vi "+S2C_VAR_Manager.vi"() -> ()   [LabVIEW 2015]
panel:
  in  "Array":T1(array[cluster])=[{"Name"="MyString", "Array"=["", "String"], "Tag"="MyString", "Indent"=0}, {"Name"="MyNumber", "Array"=["0", "Number"], "Tag"="MyNumber", "Indent"=0}, {"Name"="MyBoolean", "Array"=["False", "Boolean"], "Tag"="MyBoolean", "Indent"=0}, {"Name"="MyThis", "Array"=["", "String"], "Tag"="MyThis", "Indent"=0}, {"Name"="MyThat", "Array"=["", "String"], "Tag"="MyThat", "Indent"=0}, {"Name"="<Right-click for new variable>", "Array"=[], "Tag"="*New", "Indent"=0}]
  out "Init":bool
  out "Error Out":errorcluster
  in  "Error In":errorcluster
  in  "Table":string[](tree) caption="Variable Manager"
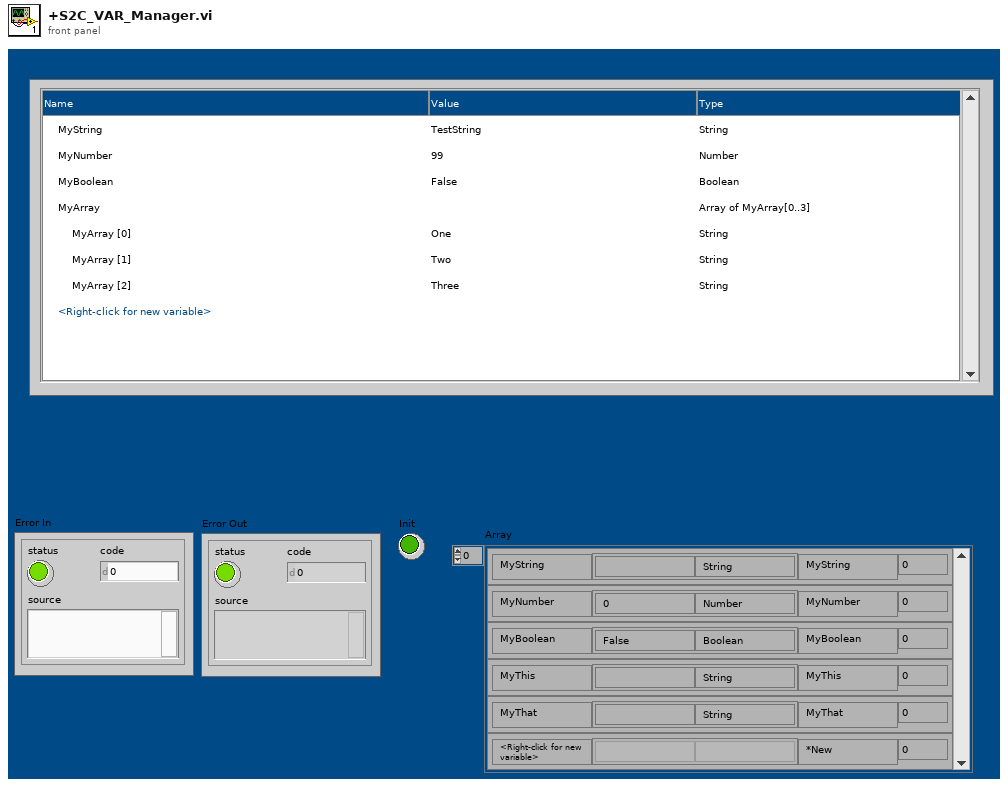
[diagram p1: front panel]
types:
  T1 = cluster{"Name":string, "Array":string[], "Tag":string, "Indent":i32}[]
  T2 = typedef "LVPoint32TypeDef.ctl" = cluster{"Horizontal":i32, "Vertical":i32}
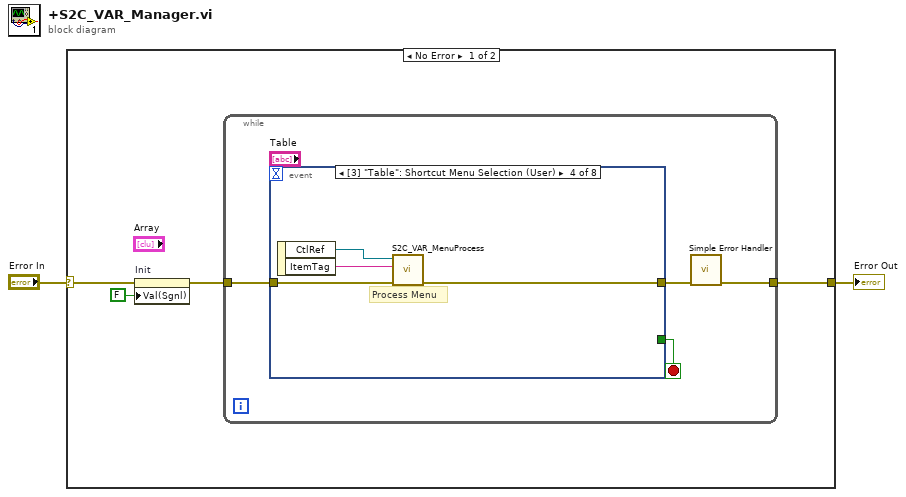
[diagram p0: block diagram]
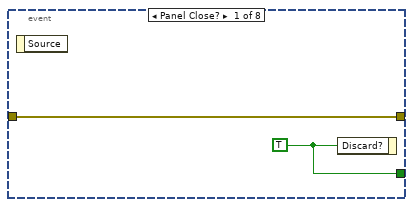
[diagram p2: hidden frame]
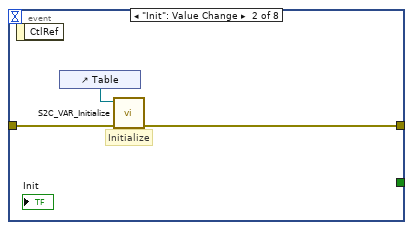
[diagram p3: hidden frame]
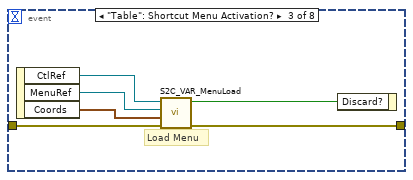
[diagram p4: hidden frame]
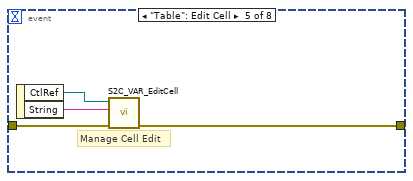
[diagram p5: hidden frame]
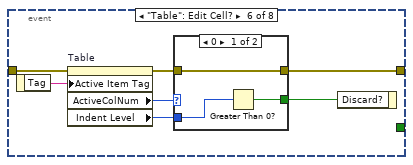
[diagram p6: hidden frame]
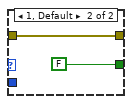
[diagram p7: hidden frame]
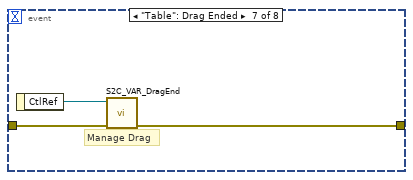
[diagram p8: hidden frame]
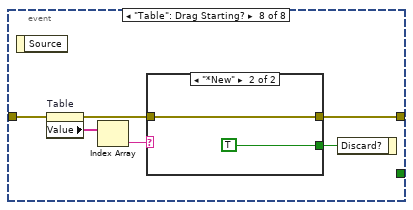
[diagram p9: hidden frame]
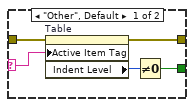
[diagram p10: hidden frame]
diagram:
  n1 = case shown="No Error" "Error In" {
    selector: "Error In" -> [w3 w58]
    tunnel: [w6 w58] -> w1
    frame No Error {
      n2 = property on="Init" class="Bool (strict)"(error in=w3, "Val(Sgnl)"=FALSE ("Value (Signaling)")) -> (error out=w5:errorcluster)  [unwired: 1 in, 1 out]
      n3 = while {
        tunnel: w5 -> [w10]
        tunnel: [w7] -> w6
        stop <- w8 stop-if-true
        n4 = event shown="[3] \"Table\": Shortcut Menu Selection (User)" {
          selector: _ -> [_ _ _ _ _ _ _ _]
          dyn-events: _ -> [_ _ _ _ _ _ _ _]
          timeout: _ -> [_ _ _ _ _ _ _ _]
          tunnel: w10 -> [w12 w15 w21 w24 w27 w36 w44 w50]
          tunnel: [w12 w13 w18 w22 w28 w31 w43 w47] -> w9
          tunnel: [w11 _ _ _ _ _ _ _] -> w8
          event Panel Close? {
            w11 = TRUE
            n5 = event-data() -> ()  [unwired: 1 in, 1 out]
            n6 = event-data("Discard?"=w11) -> ()  [unwired: 1 in, 1 out]
          }
          event "Init": Value Change {
            # "Initialize"
            n7 = event-data() -> ()  [unwired: 1 in, 1 out]
            n8 = control-ref of="Table"() -> (w14:refnum<vi>)
            n9 = call "S2C_VAR_Initialize.vi"("Error In"=w15, "CtrlRef"=w14) -> ("Error Out"=w13:errorcluster)  [unwired: 9 in]
          }
          event "Table": Shortcut Menu Activation? {
            # "Load Menu"
            n10 = event-data() -> ("CtlRef"=w16:refnum<vi>, "MenuRef"=w17:refnum<k9>, "Coords"=w20:T2)  [unwired: 1 in]
            n11 = call "S2C_VAR_MenuLoad.vi"("Error In"=w21, "Coords"=w20, "MenuRef"=w17, "CtrlRef"=w16) -> ("Error Out"=w18:errorcluster, "Discard?"=w19:bool)  [unwired: 6 in]
            n12 = event-data("Discard?"=w19) -> ()  [unwired: 1 in, 1 out]
          }
          event "Table": Shortcut Menu Selection (User) {
            # "Process Menu"
            n13 = event-data() -> ("CtlRef"=w25:refnum<vi>, "ItemTag"=w23:string)  [unwired: 1 in]
            n14 = call "S2C_VAR_MenuProcess.vi"("Error In"=w24, "ItemTag"=w23, "CtrlRef"=w25) -> ("Error Out"=w22:errorcluster)  [unwired: 8 in]
          }
          event "Table": Edit Cell {
            # "Manage Cell Edit"
            n15 = event-data() -> ("CtlRef"=w26:refnum<vi>, "String"=w29:string)  [unwired: 1 in]
            n16 = call "S2C_VAR_EditCell.vi"("Error In"=w27, "String"=w29, "CtrlRef"=w26) -> ("Error Out"=w28:errorcluster)  [unwired: 8 in]
          }
          event "Table": Edit Cell? {
            n17 = event-data() -> ("Tag"=w35:string)  [unwired: 1 in]
            n18 = property on="Table" class="Tree (strict)"(error in=w36, "Active Item Tag"=w35) -> (error out=w33:errorcluster, "ActiveColNum"=w34:i32, "Indent Level"=w32:i32)  [unwired: 1 in, 1 out]
            n19 = case shown="0" w34 {
              tunnel: w33 -> [w39 w41]
              tunnel: w32 -> [w38 _]
              tunnel: [w39 w41] -> w31
              tunnel: [w37 FALSE] -> w30
              frame 0 {
                n20 = Greater Than 0?(x=w38) -> (x > 0?=w37:bool)
              }
              frame 1, Default {
              }
            }
            n21 = event-data("Discard?"=w30) -> ()  [unwired: 1 in, 1 out]
          }
          event "Table": Drag Ended {
            # "Manage Drag"
            n22 = event-data() -> ("CtlRef"=w42:refnum<vi>)  [unwired: 1 in]
            n23 = call "S2C_VAR_DragEnd.vi"("Error In"=w44, "CtrlRef"=w42) -> ("Error Out"=w43:errorcluster)  [unwired: 9 in]
          }
          event "Table": Drag Starting? {
            n24 = event-data() -> ()  [unwired: 1 in, 1 out]
            n25 = property on="Table" class="Tree (strict)"(error in=w50) -> (error out=w48:errorcluster, "Value"=w49:string[])  [unwired: 1 in, 1 out]
            n26 = Index Array(array=w49) -> (element=w45:string)  [unwired: 1 in]
            n27 = case shown="\"*New\"" w45 {
              selector: w45 -> [w51 _]
              tunnel: w48 -> [w55 w57]
              tunnel: [w53 w57] -> w47
              tunnel: [w52 TRUE] -> w46
              frame "Other", Default {
                n28 = property on="Table" class="Tree (strict)"(error in=w55, "Active Item Tag"=w51) -> (error out=w53:errorcluster, "Indent Level"=w54:i32)  [unwired: 1 in, 1 out]
                n29 = Not Equal To 0?(x=w54) -> (x != 0?=w52:bool)
              }
              frame "*New" {
              }
            }
            n30 = event-data("Discard?"=w46) -> ()  [unwired: 1 in, 1 out]
          }
        }
        n31 = call <vilib>:"Simple Error Handler.vi"("error in (no error)"=w9) -> ("error out"=w7:errorcluster)  [unwired: 4 in, 4 out]
      }
    }
    frame Error {
    }
  }
  "Error Out" <- w1
